vi "Generate Random GB of Size 2014-11-10.vi"() -> ()   [LabVIEW 2010]
uses:
  <vilib>/Utility/file.llb/Write To Spreadsheet File (string).vi
panel:
  out "# of atoms":i32
  out "Expected # of atoms":i32
  out "Last Creation Time":T1={"Time to create primitives"=0, "Time to Grow to Box"=52, "Time to find subset"=55, "Time to Cleanup"=10}
  in  "Conventional Unit Cell":T2={"Structure Name"="CdTe", "Lattice vector a"=[6.615785553057252, 0.0, 0.0], "Lattice vector b"=[0.0, 6.615785553057252, 0.0], "Lattice vector c"=[0.0, 0.0, 6.615785553057252], "Atoms Array"=[{"Atom Name"="Cd", "Positions (Direct)"=[[0.0, 0.0, 0.0], [0.0, 0.5, 0.5], [0.5, 0.0, 0.5], [0.5, 0.5, 0.0]], "Positions (Cartesian)"=[[0.0, 0.0, 0.0], [0.0, 3.307892776528626, 3.307892776528626], [3.307892776528626, 0.0, 3.307892776528626], [3.307892776528626, 3.307892776528626, 0.0]]}, {"Atom Name"="Te", "Positions (Direct)"=[[0.25, 0.25, 0.25], [0.75, 0.75, 0.25], [0.75, 0.25, 0.75], [0.25, 0.75, 0.75]], "Positions (Cartesian)"=[[1.653946388264313, 1.653946388264313, 1.653946388264313], [4.96183916479294, 4.96183916479294, 1.653946388264313], [4.96183916479294, 1.653946388264313, 4.96183916479294], [1.653946388264313, 4.96183916479294, 4.96183916479294]]}], "# of atoms"=8}
  in  "Max # of Atoms":i32=4000
  in  "Edge Duplication Range":dbl=3.0
  in  "Min Seperation Distance (A)":dbl=2.0
  in  "Random Translation?":bool
  out "Structures / Minute":dbl=1.1005083219721028
  in  "Output Directory":path=path "D:/Ab-initio/RAGB"
  in  "Reduce to Repeating":T3={"Slab X"=4.6, "Slab Y"=4.0, "Tolerance (A)"=0.5, "Presorted?"=FALSE}
  out "Current Index":i32=80352
  out "# Created":i32=715
  in  "Grain Growth and Geometry":T4={"Grain 1 Length (prop)"=1.0, "Grain 2 Length (prop)"=1.0, "Max Grain Height (A)"=90.0, "Max Grain Width (A)"=90.0, "Grain 1 Start"=-0.001, "Overlap Region (A)"=0.001}
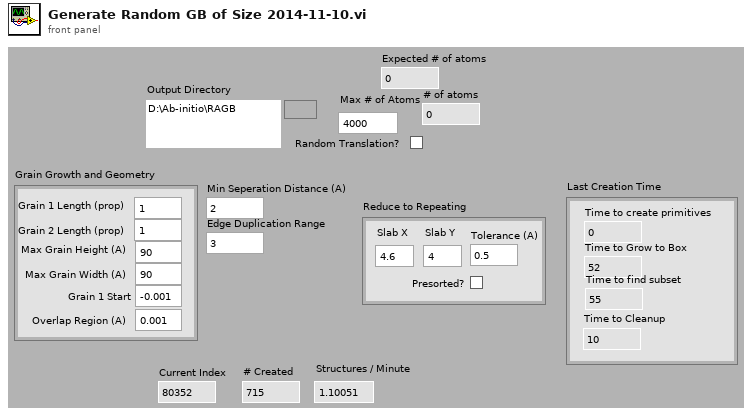
[diagram p1: front panel]
types:
  T1 = cluster{"Time to create primitives":u32, "Time to Grow to Box":u32, "Time to find subset":u32, "Time to Cleanup":u32}
  T2 = cluster{"Structure Name":string, "Lattice vector a":dbl[], "Lattice vector b":dbl[], "Lattice vector c":dbl[], "Atoms Array":cluster{"Atom Name":string, "Positions (Direct)":dbl[][], "Positions (Cartesian)":dbl[][]}[], "# of atoms":i32}
  T3 = cluster{"Slab X":dbl, "Slab Y":dbl, "Tolerance (A)":dbl, "Presorted?":bool}
  T4 = cluster{"Grain 1 Length (prop)":dbl, "Grain 2 Length (prop)":dbl, "Max Grain Height (A)":dbl, "Max Grain Width (A)":dbl, "Grain 1 Start":dbl, "Overlap Region (A)":dbl}
  T5 = cluster{"Structure Name":string, "Lattice vector a":dbl[], "Lattice vector b":dbl[], "Lattice vector c":dbl[], "Atoms Array":cluster{"Atom Name":string, "Positions (Direct)":dbl[][], "Positions (Cartesian)":dbl[][]}[], "# of atoms":i32}[]
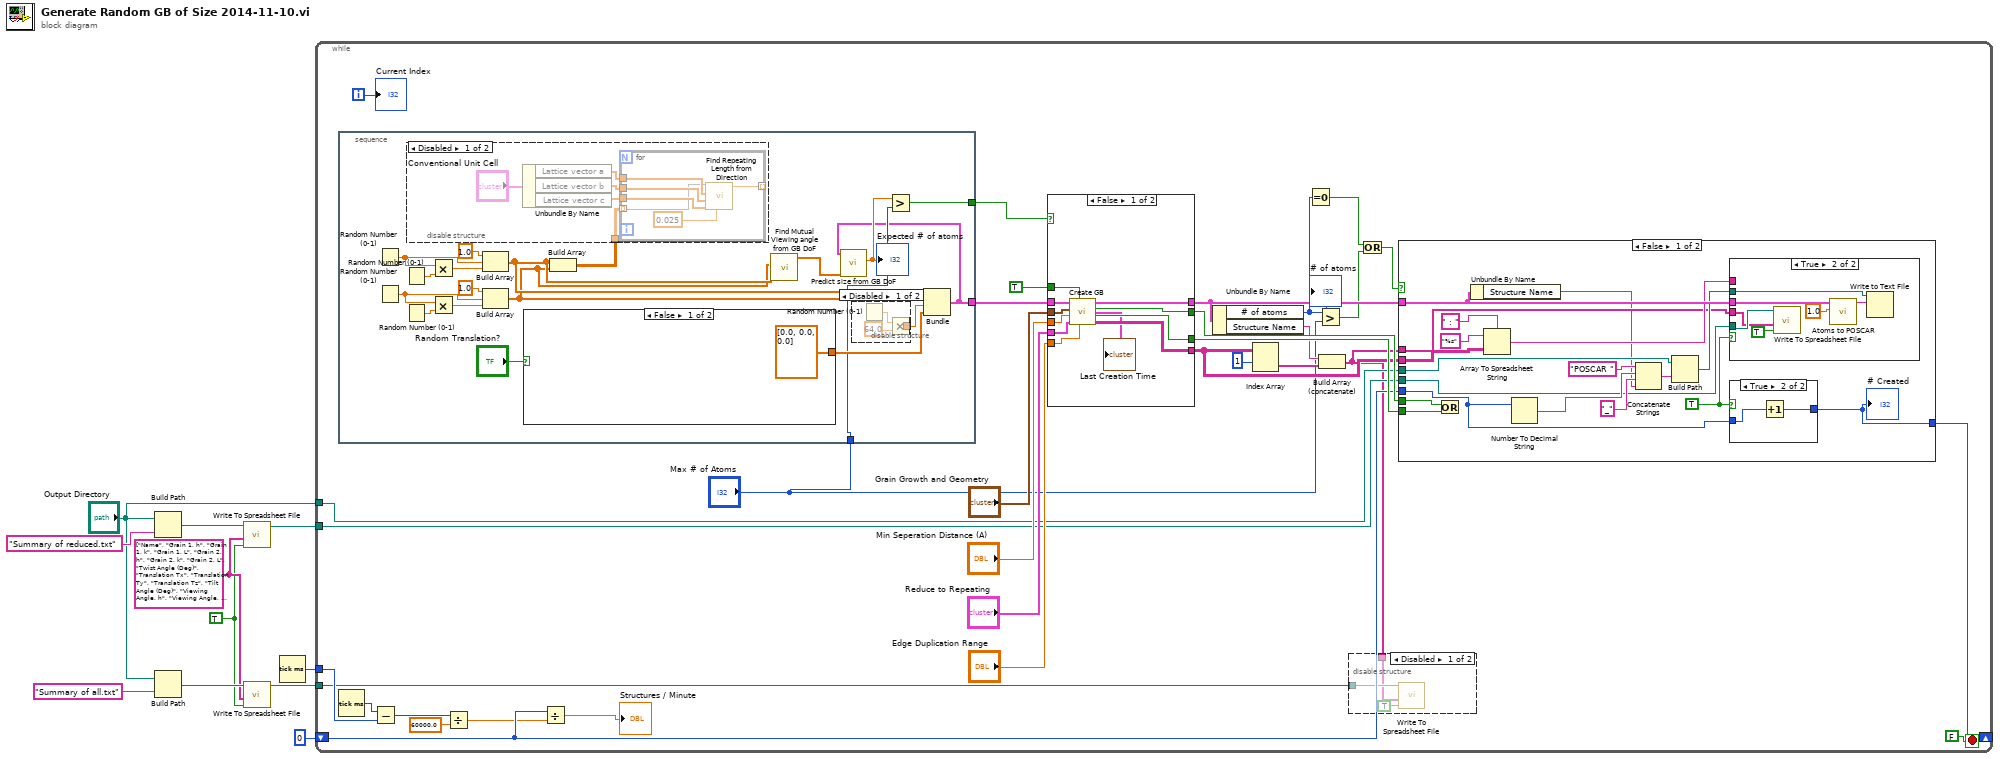
[diagram p0: block diagram]
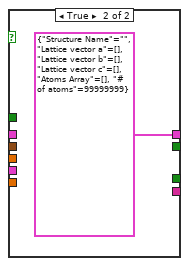
[diagram p3: hidden frame]
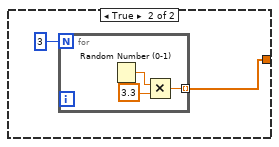
[diagram p9: hidden frame]
diagram:
  w4 = string[] ["Name", "Grain 1, h", "Grain 1, k", "Grain 1, L", "Grain 2, h", "Grain 2, k", "Grain 2, L", "Twist Angle (Deg)", "Translation Tx", "Translation Ty", "Translation Tz", "Tilt Angle (Deg)", "Viewing Angle, h", "Viewing Angle, k", "Viewing Angle, L", "Grain 1 Length (factor)", "Grain 2 Length (factor", "Max Grain Height (A)", "Max Grain Width (A)", "Grain 1 Start", "Overlap Region (A)", "Reduction Slab X", "Reduction Slab Y", "Reduction Tolerance (A)", "Min Atomic Separation Distance", "Edge Duplication Range", "# of Atoms"] ("Headers")
  w3 = TRUE ("append to file? (new file:F)")
  n1 = Build Path(base path="Output Directory", name or relative path="Summary of reduced.txt") -> (appended path=w5:path)
  n2 = Build Path(base path="Output Directory", name or relative path="Summary of all.txt") -> (appended path=w8:path)
  n3 = call-poly <vilib>:"Write To Spreadsheet File.vi"("append to file? (new file:F)"=w3, "1D data"=w4, "file path (dialog if empty)"=w5) -> ("new file path (Not A Path if cancelled)"=w2:path)  [unwired: 5 in]
  n4 = call-poly <vilib>:"Write To Spreadsheet File.vi"("append to file? (new file:F)"=w3, "1D data"=w4, "file path (dialog if empty)"=w8) -> ("new file path (Not A Path if cancelled)"=w1:path)  [unwired: 5 in]
  n5 = Tick Count (ms)() -> (millisecond timer value=w10:u32)
  n6 = while {
    shift-right: [w40] -> _
    shift-left: 0 -> [w25]
    tunnel: w10 -> [w26]
    tunnel: "Output Directory" -> [w22]
    tunnel: w2 -> [w20]
    tunnel: w1 -> [w21]
    i -> [w32]
    stop <- FALSE stop-if-true
    n7 = stacked-sequence {
      tunnel: [w90] -> w34
      tunnel: [w91] -> w27
      tunnel: "Max # of Atoms" -> [w93]
      frame #0 {
        n8 = Random Number (0-1)() -> (number: 0 to 1=w101:dbl)
        n9 = Random Number (0-1)() -> (number: 0 to 1=w105:dbl)
        n10 = Random Number (0-1)() -> (number: 0 to 1=w100:dbl)
        n11 = Random Number (0-1)() -> (number: 0 to 1=w106:dbl)
        n12 = Multiply(x=w101, y=w100) -> (x*y=w102:dbl)
        n13 = Multiply(x=w105, y=w106) -> (x*y=w107:dbl)
        n14 = Build Array(1.0 ("element"), w101, w102) -> (w95:dbl[])
        n15 = Build Array(1.0 ("element"), w105, w107) -> (w94:dbl[])
        n16 = case shown="False" "Random Translation?" {
          tunnel: [dbl[] [0.0, 0.0, 0.0] w124] -> w108
          frame False {
          }
          frame True {
            n17 = for {
              N: 3 -> [_]
              tunnel: [w126] -> w124 mode=indexing
              n18 = Random Number (0-1)() -> (number: 0 to 1=w128:dbl)
              n19 = Multiply(x=w128, y=3.3) -> (x*y=w126:dbl)
            }
          }
        }
        n20 = Build Array(w95, w94) -> (w98:dbl[][])
        n21 = disable-structure shown="Disabled" {
          disable-tunnel: w98 -> [w110 _]
          frame Disabled {
            n22 = Unbundle By Name("Conventional Unit Cell") -> ("Lattice vector a"=w111:dbl[], "Lattice vector b"=w112:dbl[], "Lattice vector c"=w113:dbl[])
            n23 = for {
              tunnel: w111 -> [w119]
              tunnel: w112 -> [w118]
              tunnel: w113 -> [w117]
              tunnel: [w115] -> _ mode=indexing
              tunnel: w110 -> [w114] mode=indexing
              n24 = call "Find Repeating Length from Direction.vi"("Tolerance"=0.025, "Lattice vector c"=w117, "Lattice vector b"=w118, "Lattice vector a"=w119, "Direction"=w114) -> ("Repeating Length (A)"=w115:dbl)  [unwired: 6 in]
            }
          }
          frame Enabled {
          }
        }
        n25 = call "Find Mutual Viewing angle from GB DoF.vi"("Viewing Angle Tolerance (Deg)"=w94, "Grain Boundary Macro DoF"=w95) -> ("Mutual Viewing Angle"=w96:dbl[])  [unwired: 7 in, 2 out]
        n26 = disable-structure shown="Disabled" {
          disable-tunnel: [w122 _] -> w97
          frame Disabled {
            n27 = Random Number (0-1)() -> (number: 0 to 1=w120:dbl)
            n28 = Multiply(x=w120, y=64.0) -> (x*y=w122:dbl)
          }
          frame Enabled {
          }
        }
        n29 = Bundle(w95, w94, w97, w108) -> (w90:cluster{dbl[], dbl[], dbl, dbl[]})  [unwired: 1 in]
        n30 = call "Predict size from GB DoF.vi"("Integer Tolerance"=w96, "Grain Boundary Definition"=w90) -> ("Expected Volume (A3)"=w92:dbl)  [unwired: 7 in, 2 out]
        "Expected # of atoms" <- w92
        n31 = Greater?(x=w92, y=w93) -> (0:w91:bool)
      }
    }
    n32 = Tick Count (ms)() -> (millisecond timer value=w28:u32)
    n33 = Subtract(x=w28, y=w26) -> (x-y=w30:u32)
    n34 = Divide(x=w30, y=60000.0) -> (x/y=w24:dbl)
    n35 = Divide(x=w25, y=w24) -> (x/y=→"Structures / Minute":dbl)
    n36 = case shown="False" w27 {
      tunnel: "Min Seperation Distance (A)" -> [w58 _]
      tunnel: "Reduce to Repeating" -> [w57 _]
      tunnel: [w56 _] -> w42
      tunnel: [w55 _] -> w41
      tunnel: TRUE ("Skip crop if no subset") -> [w54 _]
      tunnel: "Edge Duplication Range" -> [w53 _]
      tunnel: "Grain Growth and Geometry" -> [w52 _]
      tunnel: [w51 _] -> w36
      tunnel: w34 -> [w50 _]
      tunnel: [w49 T2 {"Structure Name"="", "Lattice vector a"=[], "Lattice vector b"=[], "Lattice vector c"=[], "Atoms Array"=[], "# of atoms"=99999999} ("Grain Boundary")] -> w33
      frame False {
        n37 = call "Create GB.vi"("Edge Duplication Range"=w53, "Skip cleanup if no subset"=w54, "Reduce to Repeating"=w57, "Min Seperation Distance (A)"=w58, "Grain Growth and Geometry"=w52, "Grain Boundary Definition"=w50) -> ("GB Data"=w51:string[][], "Reduced Orthorhombic?"=w55:bool, "Reduced Rhombahedral?"=w56:bool, "Grain Boundary"=w49:T2, "Ortho and Rhom"=→"Last Creation Time":T5)  [unwired: 1 in]
      }
      frame True {
      }
    }
    n38 = Unbundle By Name(w33) -> ("# of atoms"=w15:i32, "Structure Name"=w17:string)
    "# of atoms" <- w15
    n39 = Index Array(array=w36, index (row)=1) -> (element=w19:string[])  [unwired: 1 in]
    n40 = Equal To 0?(x=w15) -> (x = 0?=w14:bool)
    n41 = Greater?(x=w15, y="Max # of Atoms") -> (0:w16:bool)
    n42 = Build Array (concatenate)(w17, w19) -> (w18:string[])
    n43 = disable-structure shown="Disabled" {
      disable-tunnel: w21 -> [w47 _]
      disable-tunnel: w18 -> [w46 _]
      frame Disabled {
        n44 = call-poly <vilib>:"Write To Spreadsheet File.vi"("append to file? (new file:F)"=TRUE, "1D data"=w46, "file path (dialog if empty)"=w47) -> ()  [unwired: 5 in, 1 out]
      }
      frame Enabled {
      }
    }
    n45 = Or(x=w14, y=w16) -> (x .or. y?=w13:bool)
    n46 = case shown="False" w13 {
      tunnel: w42 -> [w78 _]
      tunnel: w41 -> [w77 _]
      tunnel: w25 -> [w61 w89]
      tunnel: [w76 w89] -> w40
      tunnel: w36 -> [w75 _]
      tunnel: w33 -> [w74 _]
      tunnel: w18 -> [w66 _]
      tunnel: w22 -> [w65 _]
      tunnel: w20 -> [w60 _]
      frame False {
        w62 = TRUE
        n47 = Or(x=w78, y=w77) -> ()  [unwired: 1 out]
        n48 = Unbundle By Name(w74) -> ("Structure Name"=w63:string)
        n49 = Array To Spreadsheet String(delimiter (Tab)=" : ", array=w75, 3:"%s" ("format string")) -> (spreadsheet string=w68:string)
        n50 = Number To Decimal String(number=w61) -> (decimal integer string=w73:string)  [unwired: 1 in]
        n51 = Concatenate Strings("POSCAR " ("string"), w73, "_" ("string"), w63) -> (w72:string)
        n52 = Build Path(base path=w65, name or relative path=w72) -> (appended path=w71:path)
        n53 = case shown="True" w62 {
          tunnel: w74 -> [_ w83]
          tunnel: w71 -> [_ w85]
          tunnel: w68 -> [_ _]
          tunnel: w66 -> [_ w79]
          tunnel: w60 -> [_ w84]
          frame False {
          }
          frame True {
            n54 = call-poly <vilib>:"Write To Spreadsheet File.vi"("append to file? (new file:F)"=TRUE, "1D data"=w79, "file path (dialog if empty)"=w84) -> ()  [unwired: 5 in, 1 out]
            n55 = call "Atoms to POSCAR.vi"("Volume Factor"=1.0, "Atomic Structure"=w83) -> ("POSCAR File"=w82:string)  [unwired: 9 in]
            n56 = Write to Text File(file (use dialog)=w85, text=w82) -> ()  [unwired: 2 in, 3 out]
          }
        }
        n57 = case shown="True" w62 {
          tunnel: w61 -> [w86 w88]
          tunnel: [w86 w87] -> w76
          frame False {
          }
          frame True {
            n58 = Increment(x=w88) -> (x+1=w87:i32)
          }
        }
        "# Created" <- w76
      }
      frame True {
      }
    }
    "Current Index" <- w32
  }
